vi "CRYView Pic WAIT Outing.vi"(8 "pVIRef":refnum<vi>, 9 "sData":string) -> (1 "sData_Out":string)   [LabVIEW 2013]
uses:
  CRYView Global.vi
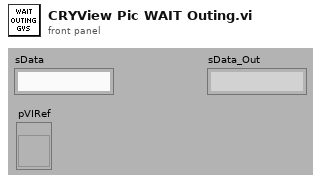
[diagram p1: front panel]
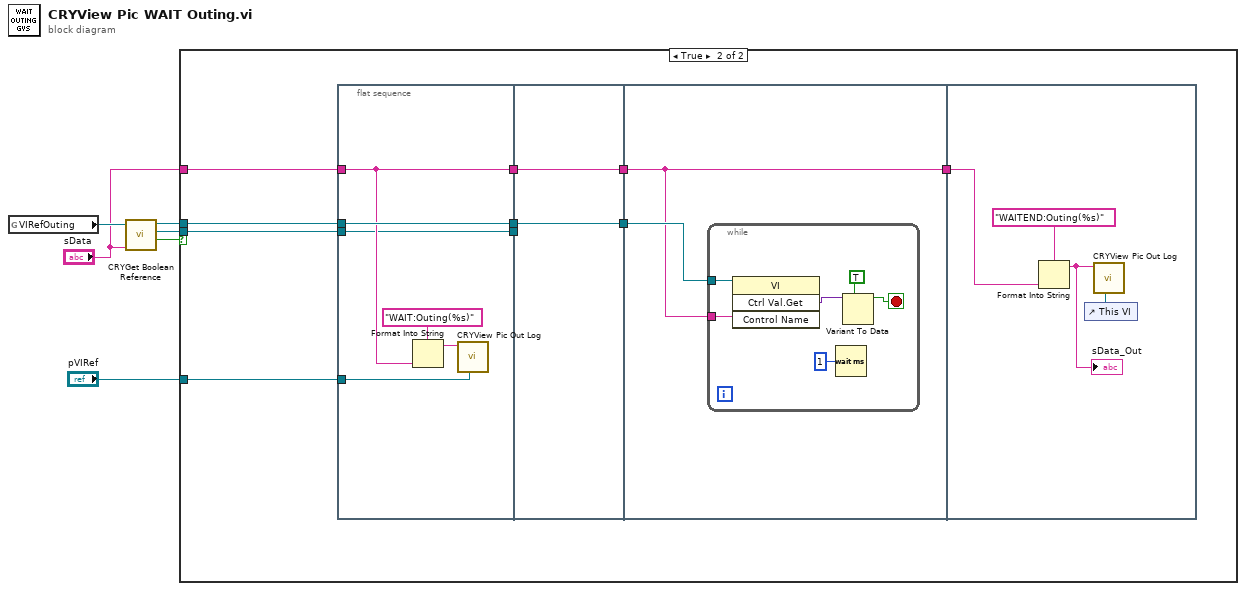
[diagram p0: block diagram]
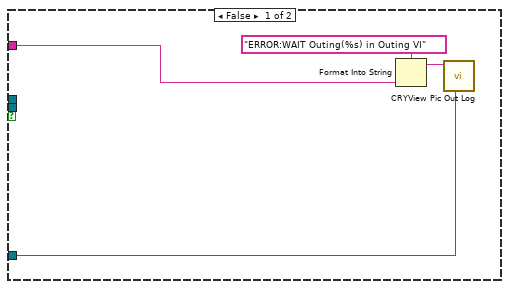
[diagram p2: hidden frame]
diagram:
  n1 = global read "CRYView Global.vi" "VIRefOuting"() -> (w5:refnum<vi>)
  n2 = call "CRYGet Boolean Reference.vi"("Label Name"="sData", "VI Refnum"=w5) -> ("Exist?"=w4:bool, "Boolean Ref"=w3:refnum<vi>, "VI Refnum Out"=w6:refnum<vi>)  [unwired: 7 in]
  n3 = case shown="True" w4 {
    tunnel: w6 -> [_ w19]
    tunnel: "pVIRef" -> [w8 w18]
    tunnel: "sData" -> [w7 w17]
    tunnel: w3 -> [_ w16]
    frame False {
      n4 = Format Into String(format string="ERROR:WAIT Outing(%s) in Outing VI" ("string"), w7) -> (resulting string=w9:string)  [unwired: 2 in, 1 out]
      n5 = call "CRYView Pic Out Log.vi"("vi reference"=w8, "sData"=w9) -> ()  [unwired: 10 in]
    }
    frame True {
      n6 = flat-sequence {
        tunnel: w19 -> [w25]
        tunnel: w18 -> [w23]
        tunnel: [w25] -> w15
        tunnel: [w22] -> w13
        tunnel: w17 -> [w22]
        tunnel: w16 -> [w21]
        tunnel: [w21] -> w11
        tunnel: w15 -> [w28]
        tunnel: [w28] -> w14
        tunnel: w13 -> [w27]
        tunnel: [w27] -> w12
        tunnel: w11 -> [_]
        tunnel: w14 -> [w30]
        tunnel: w12 -> [w29]
        tunnel: [w29] -> w20
        tunnel: w20 -> [w39]
        frame #0 {
          n7 = Format Into String(format string="WAIT:Outing(%s)" ("string"), w22) -> (resulting string=w24:string)  [unwired: 2 in, 1 out]
          n8 = call "CRYView Pic Out Log.vi"("vi reference"=w23, "sData"=w24) -> ()  [unwired: 10 in]
        }
        frame #1 {
        }
        frame #2 {
          n9 = while {
            tunnel: w30 -> [w36]
            tunnel: w29 -> [w31]
            stop <- w33 stop-if-true
            n10 = invoke class="VI" method="Ctrl Val.Get"(reference=w36, "Control Name"=w31) -> ("Get Control Value Variant"=w35:variant)  [unwired: 2 in, 3 out]
            n11 = Wait (ms)(milliseconds to wait=u32 1) -> ()  [unwired: 1 out]
            n12 = Variant To Data(type=TRUE, Variant=w35) -> (data=w33:bool)  [unwired: 1 in, 1 out]
          }
        }
        frame #3 {
          n13 = Format Into String(format string="WAITEND:Outing(%s)" ("string"), w39) -> (resulting string=w37:string)  [unwired: 2 in, 1 out]
          "sData_Out" <- w37
          n14 = control-ref of="This VI"() -> (w38:refnum<vi>)
          n15 = call "CRYView Pic Out Log.vi"("vi reference"=w38, "sData"=w37) -> ()  [unwired: 10 in]
        }
      }
    }
  }
